vi "NanotecSMCPDDriver.reset position error.vi"(0 "VISA resource name":refnum<visa-resource-name>, 1 "contollerID":i32=-1, 5 "error in (no error)":errorcluster) -> (14 "VISA resource name out":refnum<visa-resource-name>, 15 "contollerID out":i32=-1, 19 "error out":errorcluster)   [LabVIEW 2014, in "NanotecSMCPDDriver.lvlib"]
doc: "Resets the position error flag, if it is raised."
uses:
  NanotecSMCPDDriver.lvlib
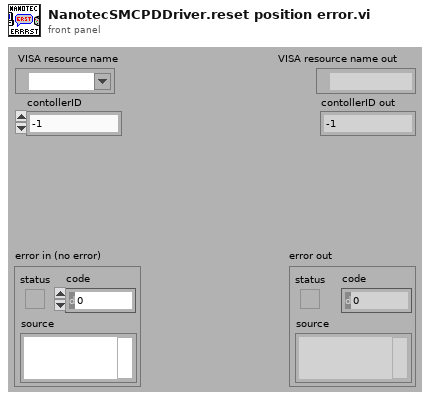
[diagram p1: front panel]
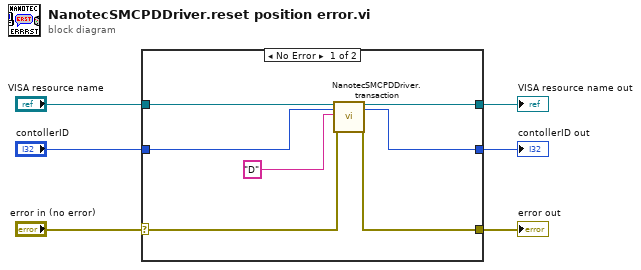
[diagram p0: block diagram]
diagram:
  n1 = case shown="No Error" "error in (no error)" {
    selector: "error in (no error)" -> [w8 w14]
    tunnel: [w10 w16] -> w6
    tunnel: [w9 w14] -> w5
    tunnel: "VISA resource name" -> [w13 w16]
    tunnel: "contollerID" -> [w12 w15]
    tunnel: [w11 w15] -> w2
    frame No Error {
      n2 = call "NanotecSMCPDDriver.transaction.vi"("VISAresource"=w13, "contollerID"=w12, "commandString"="D", "error in (no error)"=w8) -> ("VISAresource out"=w10:refnum<visa-resource-name>, "contollerID out"=w11:i32, "error out"=w9:errorcluster)  [unwired: 10 in, 3 out]
    }
    frame Error {
    }
  }
  "VISA resource name out" <- w6
  "error out" <- w5
  "contollerID out" <- w2
